vi "Get Provided Interface.vi"(8 "error in":errorcluster, 11 "instrument in":refnum<class "Instrument.lvclass">) -> (0 "error out":errorcluster, 2 "provided interface":string, 3 "instrument out":refnum<class "Instrument.lvclass">)   [LabVIEW 2020, in "MeasurementLink niFGEN.lvlib" / "Instrument.lvclass"]
uses:
  Instrument.lvclass
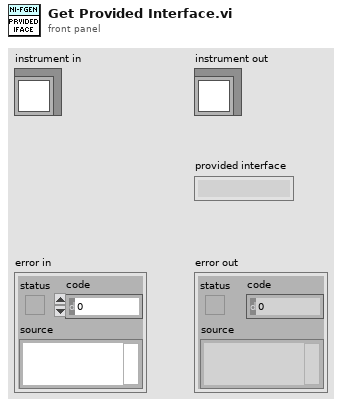
[diagram p1: front panel]
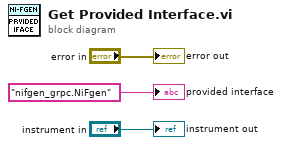
[diagram p0: block diagram]
diagram:
  "error out" <- "error in"
  "instrument out" <- "instrument in"
  "provided interface" <- "nifgen_grpc.NiFgen" ("provided interface")
